vi "solar Build INI Path.vi"(10 "Name":string, 11 "solar in":refnum<class "solar.lvclass">) -> (2 "appended path":path, 3 "solar out":refnum<class "solar.lvclass">)   [LabVIEW 2018, in "solar.lvclass"]
doc: "This function builds an ini path for a specified target."
uses:
  solar.lvclass
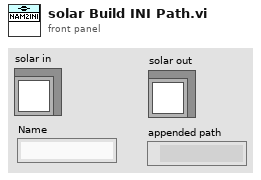
[diagram p1: front panel]
types:
  T1 = typedef "solar_ctl SOLAR Refnum.ctl" = refnum<k1>
  T2 = typedef "solar_ctl SOLAR Global.ctl" = cluster{"Targets":T3[], "AppDir":path, "solar.ini":path, "ConfigsDir":path, "CosmosDir":path, "LogsDir":path, "ExePath":path, "ExeVersion":string, "PartNum":string, "AppSetup":string, "Title":string, "Main.ini":path, "Temp.ini":path, "vSOLAR":string, "Splash.png":string, "SplashWait":i32, "SOLARUE":refnum<user-event>, "VoyagerRefnum":T4, "QTimerRefnum":T5}
  T3 = typedef "solar_ctl Target Global.ctl" = cluster{"Target":string, "Q":refnum<queue>, "UE":refnum<user-event>, "VI":refnum<vi>, "Menu":refnum<k9>, "Data":refnum<data-value>, "Attributes":variant}
  T4 = typedef "solar_voy_ctl Voyager Refnum.ctl" = refnum<k1>
  T5 = typedef "solar_qtimer_ctl Refnum.ctl" = refnum<k1>
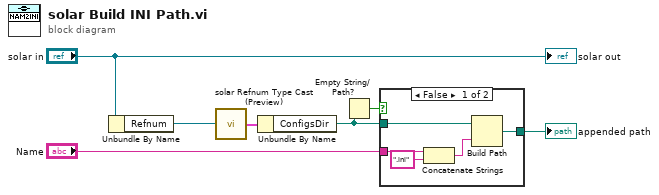
[diagram p0: block diagram]
diagram:
  n1 = Unbundle By Name("solar in") -> ("Refnum"=w1:T1)
  n2 = call "solar Refnum Type Cast (Preview).vi"("Refnum"=w1) -> ("SOLAR"=w6:T2)  [unwired: 8 in]
  n3 = Unbundle By Name(w6) -> ("ConfigsDir"=w4:path)
  n4 = Empty String/Path?(string/path=w4) -> (empty?=w5:bool)
  n5 = case shown="False" w5 {
    tunnel: "Name" -> [w12 _]
    tunnel: w4 -> [w10 _]
    tunnel: [w8 _] -> w3
    frame False {
      n6 = Concatenate Strings(w12, ".ini" ("string")) -> (w9:string)
      n7 = Build Path(base path=w10, name or relative path=w9) -> (appended path=w8:path)
    }
    frame True {
    }
  }
  "appended path" <- w3
  "solar out" <- "solar in"
